vi "Build and Parse Write Message.vi"(0 "Write Data In [DUT Ordered]":u8[][](array[numeric]) format="%02x", 1 "Message In":string, 5 "Socket Mask [U32] In":u32=1 format="%06x", 7 "Cycle Mode In":bool, 11 "error in":errorcluster) -> (3 "Message Out":string, 4 "Write Data Out [DUT Ordered]":u8[][](array[numeric]) format="%02x", 6 "Socket Mask [U32] Out":u32=1 format="%06x", 8 "Cycle Mode Out":bool, 14 "Byte Count":u8, 15 "error out":errorcluster)   [LabVIEW 2017, in "Host SRL.lvlib"]
uses:
  Host SRL.lvlib
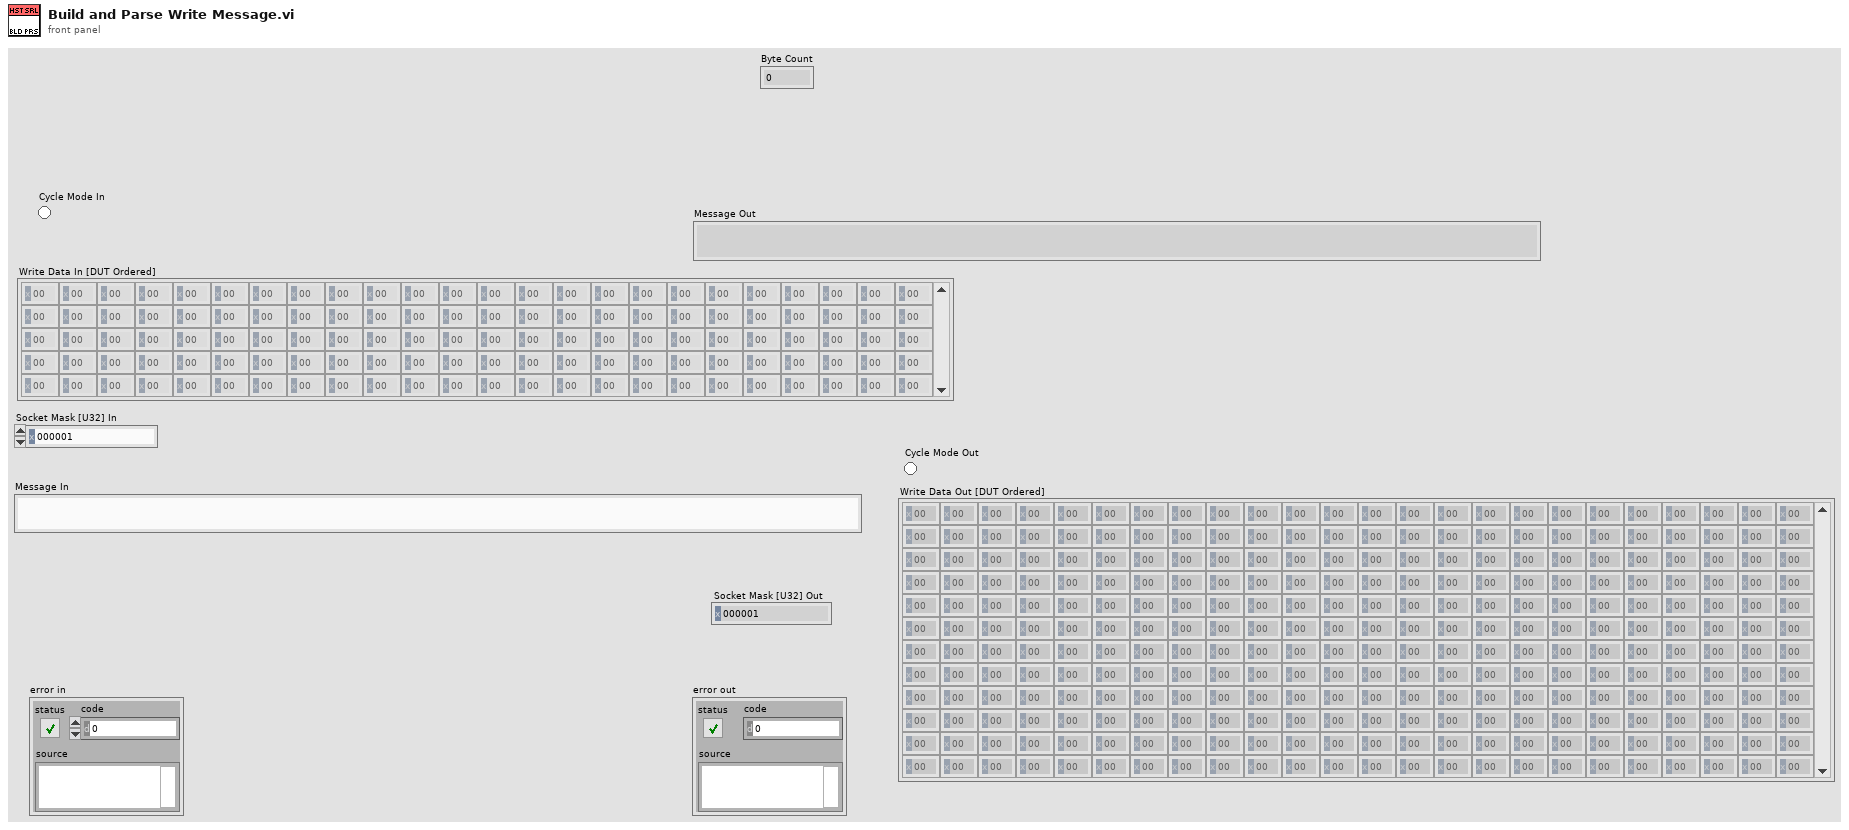
[diagram p1: front panel]
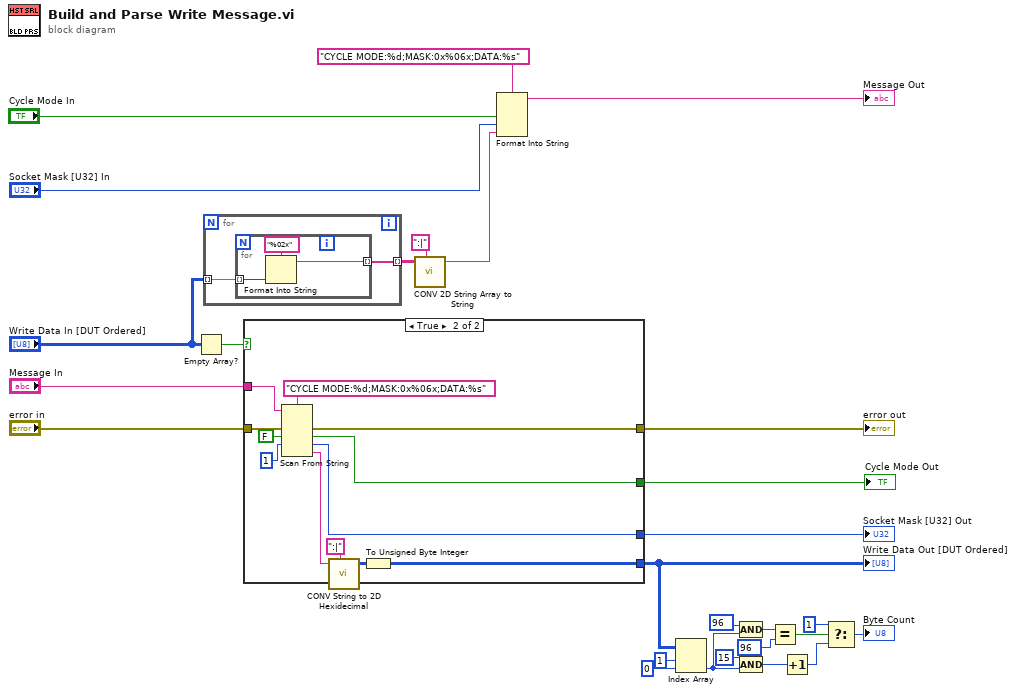
[diagram p0: block diagram]
diagram:
  n1 = Empty Array?(array="Write Data In [DUT Ordered]") -> (empty?=w20:bool)
  n2 = for {
    tunnel: "Write Data In [DUT Ordered]" -> [w29] mode=indexing
    tunnel: [w28] -> w18 mode=indexing
    n3 = for {
      tunnel: w29 -> [w32] mode=indexing
      tunnel: [w31] -> w28 mode=indexing
      n4 = Format Into String(format string="%02x", w32) -> (resulting string=w31:string)  [unwired: 2 in, 1 out]
    }
  }
  n5 = case shown="True" w20 {
    tunnel: [_ w44] -> w12
    tunnel: [_ w42] -> w25
    tunnel: "error in" -> [w33 w40]
    tunnel: [w33 w39] -> w23
    tunnel: "Message In" -> [_ w37]
    tunnel: [_ w34] -> w1
    frame False {
    }
    frame True {
      n6 = Scan From String(format string="CYCLE MODE:%d;MASK:0x%06x;DATA:%s", input string=w37, error in=w40, default 1=FALSE ("Cycle Mode"), default 2=u32 1 ("Socket Mask [U16] Out")) -> (error out=w39:errorcluster, output 1=w34:bool, output 2=w42:u32, output 3=w41:string)  [unwired: 2 in, 2 out]
      n7 = call "CONV String to 2D Hexidecimal.vi"("String"=w41, "Delimiters (,;)"=":|") -> ("2-D Hexidecimal"=w45:u32[][])  [unwired: 7 in]
      n8 = To Unsigned Byte Integer(number=w45) -> (unsigned 8bit integer=w44:u8[][])
    }
  }
  "Write Data Out [DUT Ordered]" <- w12
  "Socket Mask [U32] Out" <- w25
  "error out" <- w23
  "Cycle Mode Out" <- w1
  n9 = call "CONV 2D String Array to String.vi"("2-D String"=w18, "Delimiters (,;)"=":|") -> ("String"=w17:string)  [unwired: 7 in]
  n10 = Format Into String(format string="CYCLE MODE:%d;MASK:0x%06x;DATA:%s", "Cycle Mode In", "Socket Mask [U32] In", w17) -> (resulting string=→"Message Out":string)  [unwired: 2 in, 1 out]
  n11 = Index Array(array=w12, index (row)=1, index (col)=0 ("disabled index (col)")) -> (element=w9:u8)
  n12 = Compound Arithmetic op=AND(u8 96 ("index (row)"), w9) -> (w8:u8)
  n13 = Compound Arithmetic op=AND(u8 15 ("index (row)"), w9) -> (w13:u8)
  n14 = Equal?(x=w8, y=u8 96) -> (x = y?=w6:bool)
  n15 = Increment(x=w13) -> (x+1=w4:u8)
  n16 = Select(t=u8 1 ("Byte Count"), s=w6, f=w4) -> (s? t:f=→"Byte Count":u8)
